vi "Enable Motor.vi"(8 "Error In":errorcluster, 10 "On/Off":enum16{"On", "Off"}(ring), 11 "Address / Port":i16=1 min=1 max=31 step=1) -> (0 "Error Out":errorcluster, 3 "Address / Port dup":i16)   [LabVIEW 2014]
doc: "Set the all the motors connected to the ESP300 controller ON/OFF."
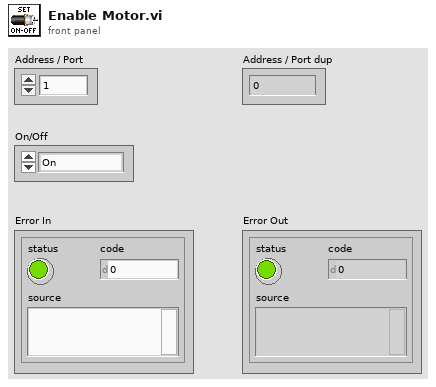
[diagram p1: front panel]
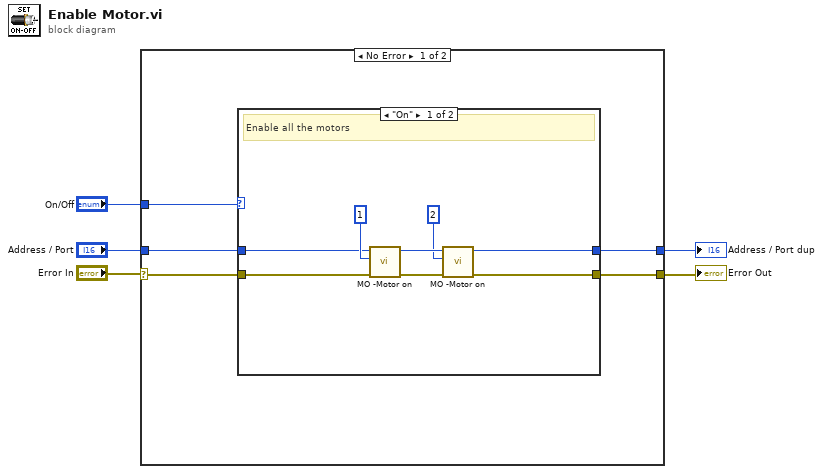
[diagram p0: block diagram]
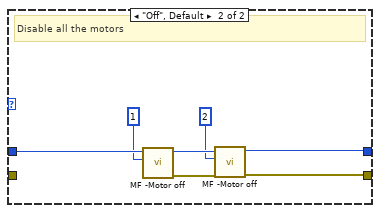
[diagram p2: hidden frame]
diagram:
  n1 = case shown="No Error" "Error In" {
    selector: "Error In" -> [w7 w26]
    tunnel: "Address / Port" -> [w10 w27]
    tunnel: [w9 w27] -> w4
    tunnel: [w8 w26] -> w3
    tunnel: "On/Off" -> [w6 _]
    frame No Error {
      n2 = case shown="\"On\"" w6 {
        tunnel: w10 -> [w14 w25]
        tunnel: [w13 w20] -> w9
        tunnel: [w12 w19] -> w8
        tunnel: w7 -> [w11 _]
        frame "On" {
          # "Enable all the motors"
          n3 = call "MO -Motor on.vi"("error in"=w11, "Axis #"=i8 1, "Address / Port"=w14) -> ("error out"=w18:errorcluster, "Address / Port dup"=w17:i16)  [unwired: 1 in, 2 out]
          n4 = call "MO -Motor on.vi"("error in"=w18, "Axis #"=i8 2, "Address / Port"=w17) -> ("error out"=w12:errorcluster, "Address / Port dup"=w13:i16)  [unwired: 1 in, 2 out]
        }
        frame "Off", Default {
          # "Disable all the motors"
          n5 = call "MF -Motor off.vi"("Axis #"=i8 1, "Address / Port"=w25) -> ("error out"=w22:errorcluster, "Address / Port dup"=w23:i16)  [unwired: 2 in, 2 out]
          n6 = call "MF -Motor off.vi"("error in"=w22, "Axis #"=i8 2, "Address / Port"=w23) -> ("error out"=w19:errorcluster, "Address / Port dup"=w20:i16)  [unwired: 1 in, 2 out]
        }
      }
    }
    frame Error {
    }
  }
  "Address / Port dup" <- w4
  "Error Out" <- w3
